vi "impedance spec.vi"(11 "Impedance Spec:":string[][](table)=[["Mating Area", "1", "110", "1", "90"], ["Cable Area", "2", "110", "2", "95"]]) -> (3 "Impedance spec string":string)   [LabVIEW 2011]
panel:
  in  "Impedance Spec String":string="1@110@2@110;1@90@2@95"
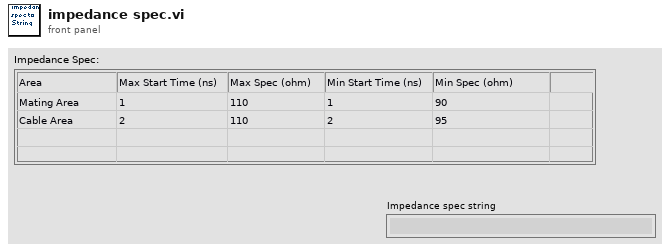
[diagram p1: front panel]
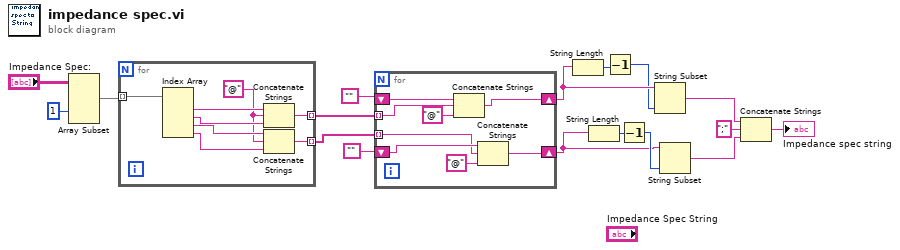
[diagram p0: block diagram]
diagram:
  n1 = Array Subset(array="Impedance Spec:", index (col)=1 ("索引")) -> (w15:string[][])  [unwired: 3 in]
  n2 = for {
    tunnel: w15 -> [w25] mode=indexing
    tunnel: [w19] -> w12 mode=indexing
    tunnel: [w18] -> w11 mode=indexing
    w21 = "@" ("字符串")
    n3 = Index Array(array=w25) -> (element #1=w24:string, element #2=w23:string, element #3=w22:string, element #4=w20:string)  [unwired: 4 in]
    n4 = Concatenate Strings(w24, w21, w23) -> (w19:string)
    n5 = Concatenate Strings(w22, w21, w20) -> (w18:string)
  }
  n6 = for {
    shift-right: [w27] -> w10
    shift-left: "" -> [w33]
    shift-right: [w26] -> w5
    shift-left: "" -> [w29]
    tunnel: w12 -> [w32] mode=indexing
    tunnel: w11 -> [w28] mode=indexing
    n7 = Concatenate Strings(w33, w32, "@" ("字符串")) -> (w27:string)
    n8 = Concatenate Strings(w29, w28, "@" ("字符串")) -> (w26:string)
  }
  n9 = String Length(string=w10) -> (length=w9:i32)
  n10 = String Length(string=w5) -> (length=w7:i32)
  n11 = Decrement(x=w9) -> (x-1=w8:i32)
  n12 = Decrement(x=w7) -> (x-1=w6:i32)
  n13 = String Subset(string=w10, length (rest)=w8) -> (substring=w4:string)  [unwired: 1 in]
  n14 = String Subset(string=w5, length (rest)=w6) -> (substring=w2:string)  [unwired: 1 in]
  n15 = Concatenate Strings(w4, ";" ("字符串"), w2) -> (→"Impedance spec string":string)
